vi "deg to rad(SubVI).vi"(1 "Degree":dbl) -> (0 "Radian":dbl)   [LabVIEW 2010]
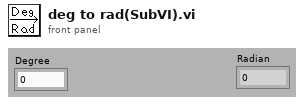
[diagram p1: front panel]
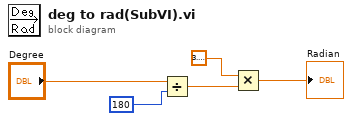
[diagram p0: block diagram]
diagram:
  n1 = Divide(x="Degree", y=180) -> (x/y=w5:dbl)
  n2 = Multiply(x=3.141592653589793, y=w5) -> (x*y=→"Radian":dbl)
